vi "Parse Data Logger Output.vi"(8 "error in":errorcluster, 11 "Data Logger Output":string) -> (0 "error out":errorcluster, 1 "Raw Data":dbl[][][](array[numeric]), 2 "Resampled Data":waveform(dbl)[](array[waveform]), 3 "Device List":string[](array[string]))   [LabVIEW 2013, in "Data Log Fetcher.lvlib"]
uses:
  Data Log Fetcher.lvlib
panel:
  # "Values for E:201VAC from 19-MAR-2015 00:00:00 to 19-MAR-2015 00:01:00 from MTA\n19-MAR-2015 00:00:00.772   1.835E-07\n1 values for E:201VAC were found from MTA"
  # "No values for E:201VAC were found in the requested time interval from node MTA."
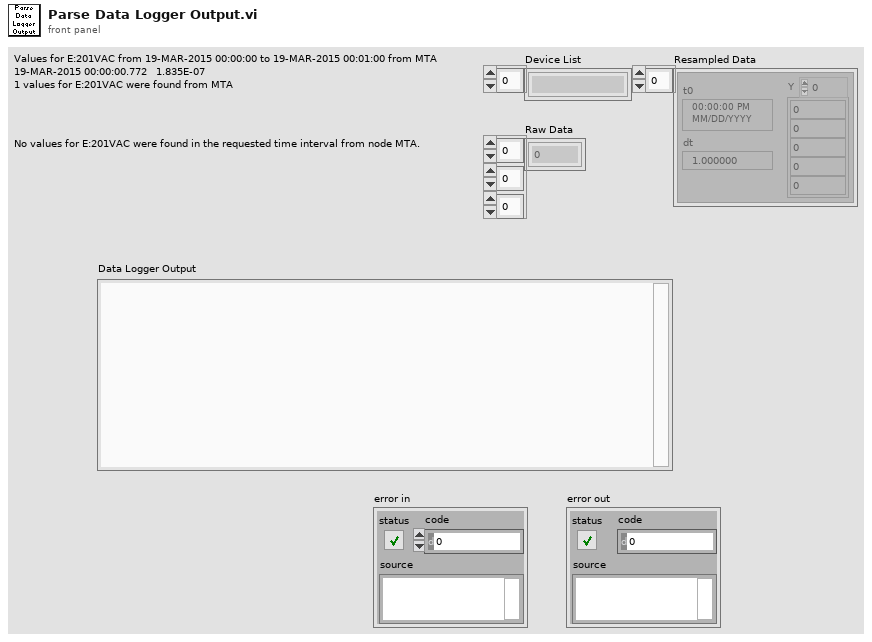
[diagram p1: front panel]
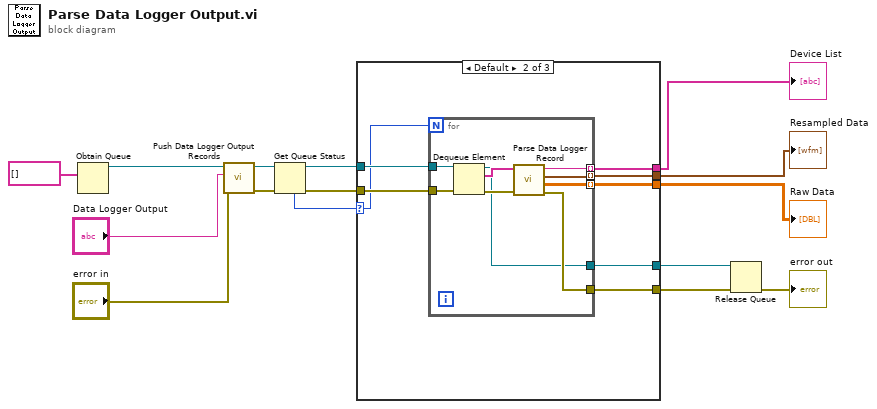
[diagram p0: block diagram]
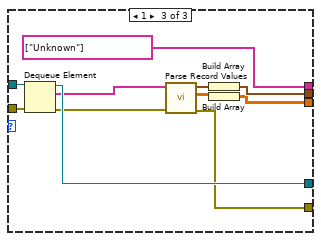
[diagram p3: hidden frame]
diagram:
  n1 = Obtain Queue(element data type=string[] []) -> (queue out=w15:refnum<queue>)  [unwired: 4 in, 2 out]
  n2 = call "Push Data Logger Output Records.vi"("error in"="error in", "Data Logger Output"="Data Logger Output", "queue in"=w15) -> ("error out"=w11:errorcluster, "queue out"=w10:refnum<queue>)  [unwired: 7 in]
  n3 = Get Queue Status(queue=w10, error in (no error)=w11) -> (queue out=w9:refnum<queue>, error out=w8:errorcluster, # elements in queue=w4:i32)  [unwired: 1 in, 5 out]
  n4 = case shown="Default" w4 {
    selector: w4 -> [_ w18 _]
    tunnel: w9 -> [w17 w25 w45]
    tunnel: w8 -> [w16 w24 w44]
    tunnel: [_ w23 string[] ["Unknown"]] -> w3
    tunnel: [_ w22 w36] -> w2
    tunnel: [_ w21 w35] -> w1
    tunnel: [w17 w20 w43] -> w7
    tunnel: [w16 w19 w42] -> w6
    frame 0 {
    }
    frame Default {
      n5 = for {
        N: w18 -> [_]
        tunnel: [w34] -> w21 mode=indexing
        tunnel: w25 -> [w31]
        tunnel: w24 -> [w30]
        tunnel: [w29] -> w23 mode=indexing
        tunnel: [w28] -> w22 mode=indexing
        tunnel: [w27] -> w19
        tunnel: [w26] -> w20
        n6 = Dequeue Element(queue=w31, error in (no error)=w30) -> (queue out=w26:refnum<queue>, element=w33:string[], error out=w32:errorcluster)  [unwired: 1 in, 1 out]
        n7 = call "Parse Data Logger Record.vi"("error in"=w32, "Record"=w33) -> ("error out"=w27:errorcluster, "Raw Data"=w34:dbl[][], "Resampled Data"=w28:waveform(dbl), "Device Name"=w29:string)  [unwired: 6 in]
      }
    }
    frame 1 {
      n8 = Dequeue Element(queue=w45, error in (no error)=w44) -> (queue out=w43:refnum<queue>, element=w41:string[], error out=w40:errorcluster)  [unwired: 1 in, 1 out]
      n9 = call "Parse Record Values.vi"("error in"=w40, "Record Values"=w41) -> ("error out"=w42:errorcluster, "Raw Data"=w37:dbl[][], "Resampled Data"=w38:waveform(dbl))  [unwired: 7 in]
      n10 = Build Array(w38) -> (w36:waveform(dbl)[])
      n11 = Build Array(w37) -> (w35:dbl[][][])
    }
  }
  "Device List" <- w3
  "Raw Data" <- w1
  "Resampled Data" <- w2
  n12 = Release Queue(queue=w7, error in (no error)=w6) -> (error out=→"error out":errorcluster)  [unwired: 1 in, 2 out]
